vi "test Loopback with Disable.vi"(8 "error in":errorcluster, 11 "TestCase in":refnum<class "Single Core Simple Loopback.lvclass">) -> (0 "error out":errorcluster, 3 "TestCase out":refnum<class "Single Core Simple Loopback.lvclass">)   [LabVIEW 2020, in "Single Core Simple Loopback.lvclass"]
uses:
  Single Core Simple Loopback.lvclass
  C:/Git/niveristand-custom-device-testing-tools/VeriStandTestCase/VeriStandTestCase.lvclass
  <vilib>/numeric/Random Number (Range) I64.vi
  2771a990-9a12-45e1-bfa9-cf8078c77ee0.vi
  97c2081a-a4c0-4f2f-8a1c-7834fbf3da42.vi
  194ce8b8-c6d7-4123-a4fb-3c321acd640d.vi
  639b215b-9681-4d6c-ae13-b880b31cf4b5.vi
  <vilib>/numeric/sub_Random U32.vi
  <vilib>/NI VeriStand/Execution/Workspace/NI VeriStand - Get Single Channel Value.vi
  <vilib>/NI VeriStand/Execution/Workspace/NI VeriStand - Set Multiple Channel Values.vi
  <vilib>/NI VeriStand/Execution/Workspace/NI VeriStand - Get Multiple Channel Values.vi
  <vilib>/addons/_JKI Toolkits/VI Tester/TestCase.llb/TestCase.lvclass
  <vilib>/NI VeriStand/Execution/Workspace/NI_VS Workspace ExecutionAPI.lvlib
  niveristand-custom-device-testing-tools/VeriStandTestUtilities/VeriStandTestUtilities.lvlib
  C:/Program Files (x86)/National Instruments/LabVIEW 2020/vi.lib/addons/_JKI Toolkits/VI Tester/TestCase.llb/TestCase.lvclass
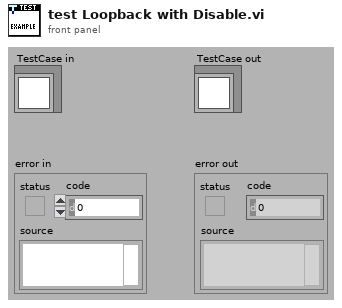
[diagram p1: front panel]
types:
  T1 = typedef "NI_VS Workspace ExecutionAPI.lvlib/WorkspaceAPI.ctl" = refnum<k24>
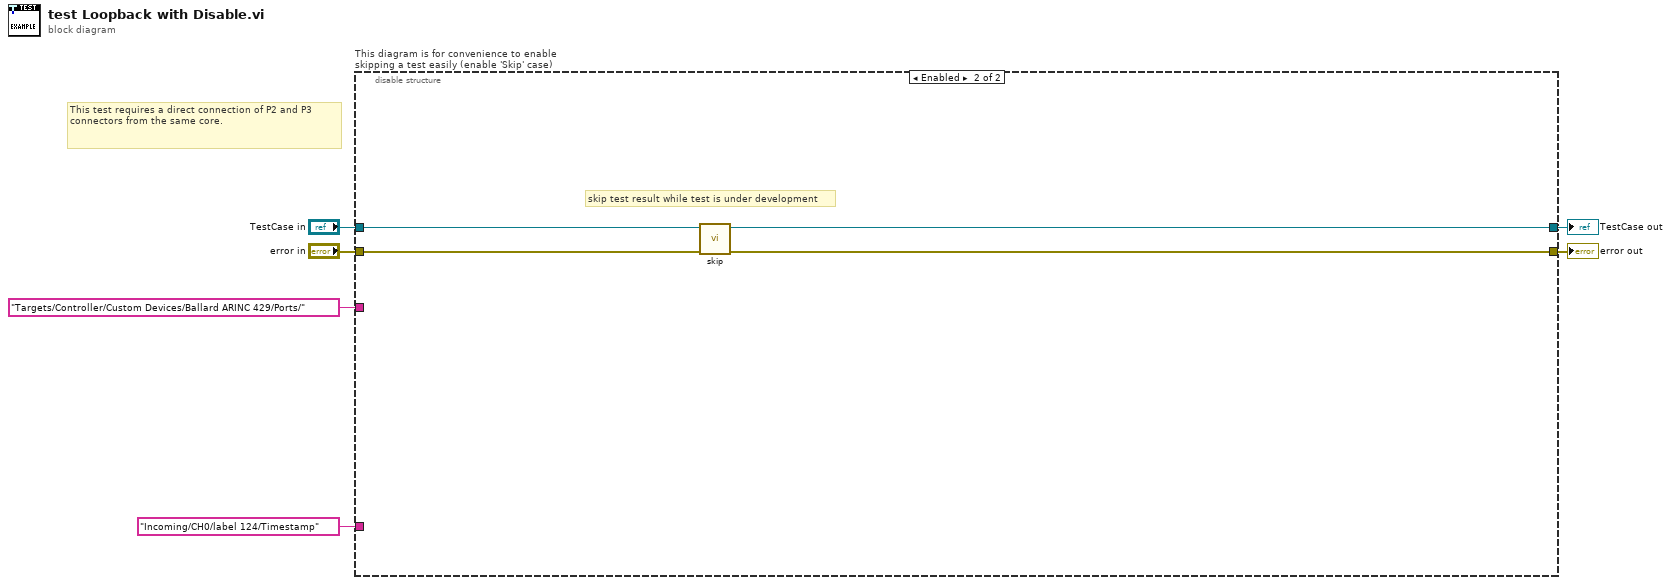
[diagram p0: block diagram]
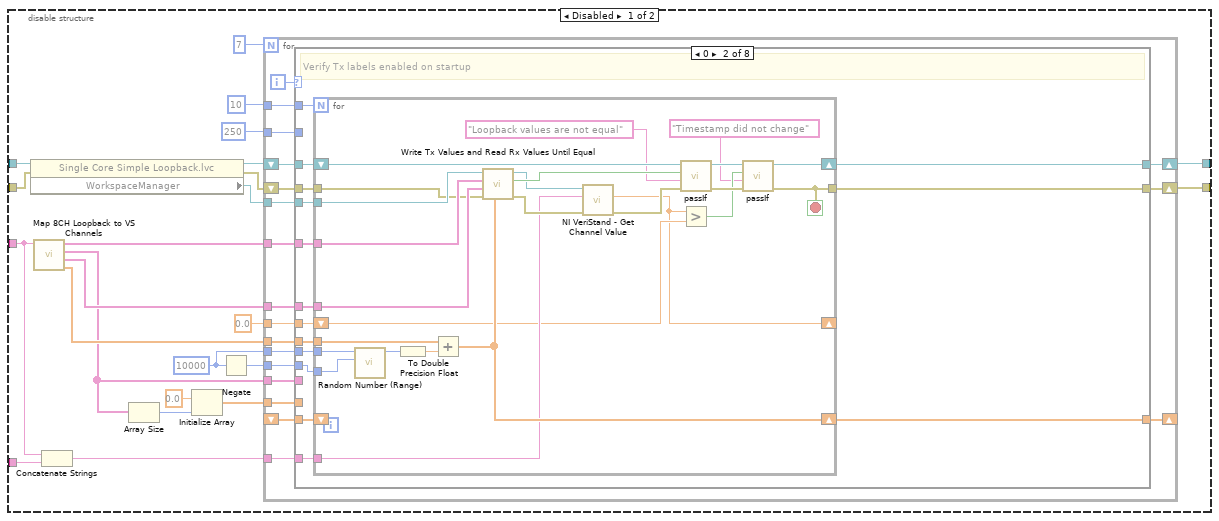
[diagram p2: hidden frame]
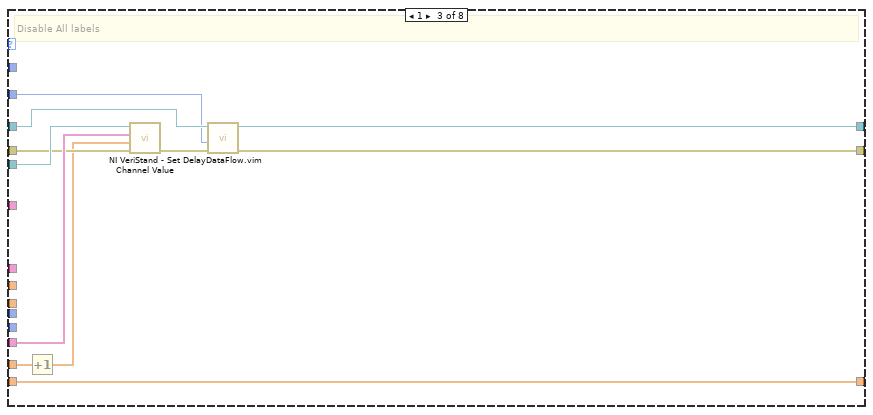
[diagram p4: hidden frame]
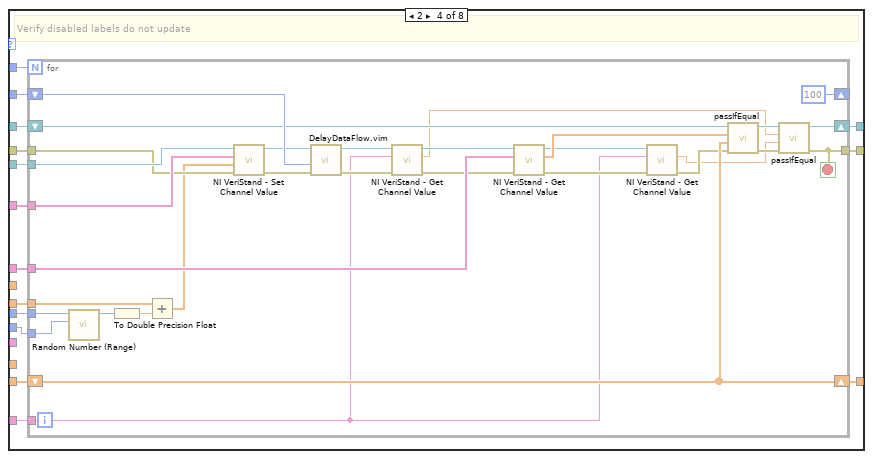
[diagram p5: hidden frame]
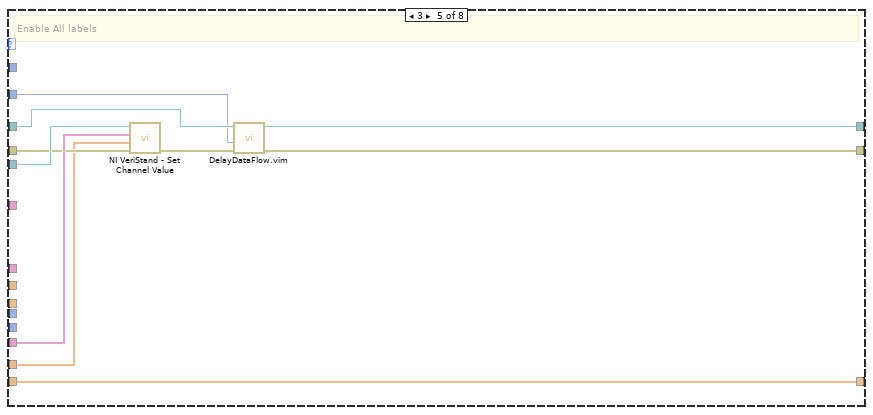
[diagram p6: hidden frame]
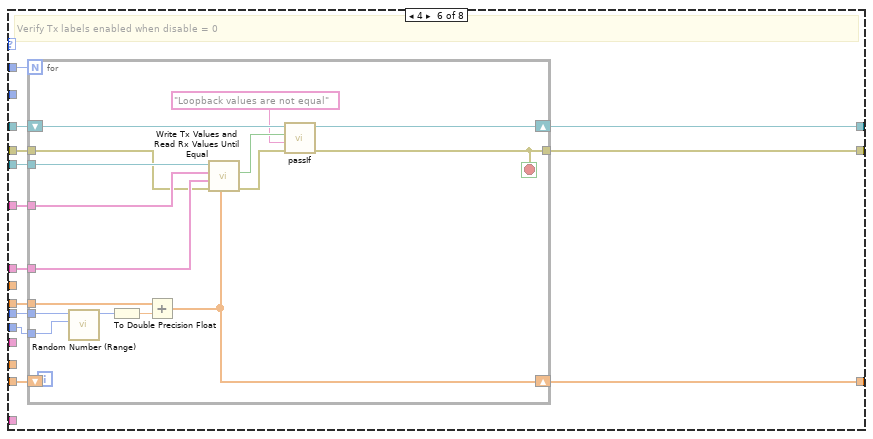
[diagram p7: hidden frame]
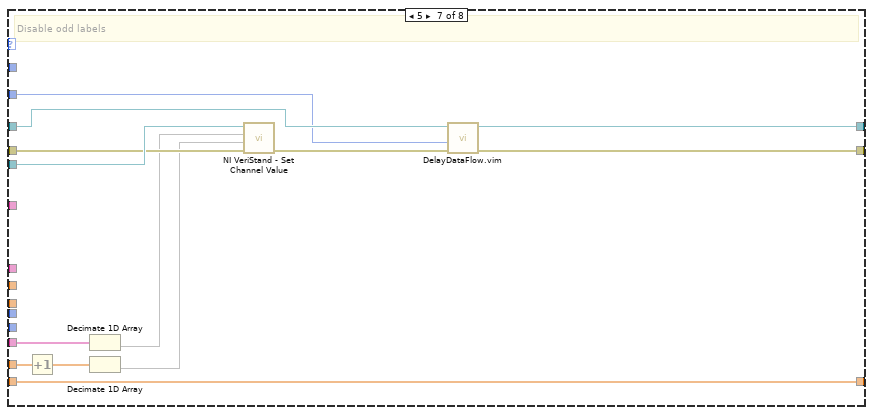
[diagram p8: hidden frame]
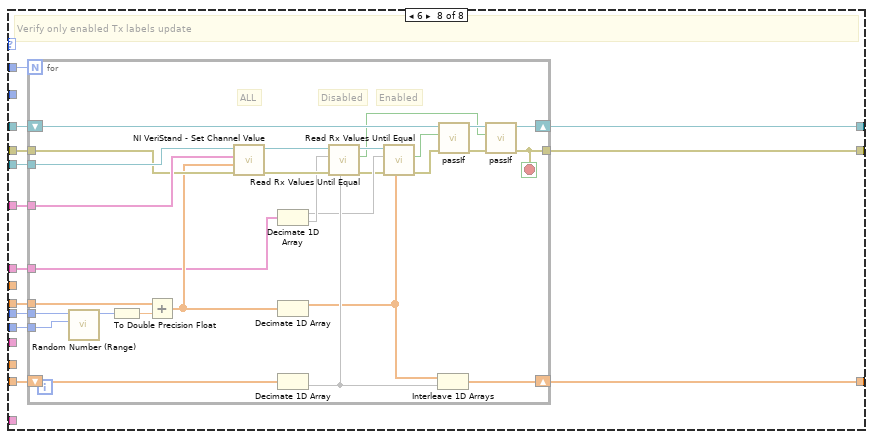
[diagram p9: hidden frame]
diagram:
  # "This test requires a direct connection of P2 and P3 connectors from the same core."
  n1 = disable-structure "This diagram is for convenience to enable skipping a test easily (enable 'Skip' case)" shown="Enabled" {
    disable-tunnel: "TestCase in" -> [w11 w241]
    disable-tunnel: [w8 w239] -> w3
    disable-tunnel: [w7 w240] -> w5
    disable-tunnel: "error in" -> [w10 w238]
    disable-tunnel: "Targets/Controller/Custom Devices/Ballard ARINC 429/Ports/" ("Channel") -> [w12 _]
    disable-tunnel: "Incoming/CH0/label 124/Timestamp" ("Channel") -> [w19 _]
    frame Disabled {
      w29 = i64 10000 ("upper bound (100)")
      n2 = property class="Single Core Simple Loopback.lvc"(reference=w11, error in=w10) -> (reference out=w25:refnum<class "Single Core Simple Loopback.lvclass">, error out=w9:errorcluster, "WorkspaceManager"=w27:T1)
      n3 = call "Map 8CH Loopback to VS Channels.vi"("Base Path to Ports"=w12) -> ("Channel Count"=w14:dbl[], "Rx Channel Array"=w15:string[], "Disable Channel Array"=w13:string[], "Tx Channel Array"=w16:string[])  [unwired: 7 in]
      n4 = Concatenate Strings(w12, w19) -> (w18:string)
      n5 = Array Size(array=w13) -> (size(s)=w24:i32)
      n6 = Initialize Array(0.0 ("element"), w24) -> (w22:dbl[])
      n7 = Negate(x=w29) -> (-x=w28:i64)
      n8 = for {
        N: 7 -> [_]
        tunnel: w14 -> [w48]
        tunnel: w29 -> [w47]
        tunnel: w28 -> [w46]
        tunnel: w16 -> [w45]
        tunnel: w27 -> [w44]
        tunnel: 10 -> [w43]
        tunnel: w15 -> [w41]
        shift-right: [w38] -> w7
        shift-left: w9 -> [w42]
        shift-right: [w39] -> w8
        shift-left: w25 -> [w40]
        tunnel: w13 -> [w36]
        tunnel: w22 -> [w35]
        shift-right: [w34] -> _
        shift-left: _ -> [w33]
        tunnel: u32 250 ("milliseconds to wait") -> [w32]
        tunnel: w18 -> [w31]
        tunnel: 0.0 ("Value") -> [w30]
        i -> [w37]
        n9 = case shown="0" w37 {
          tunnel: w48 -> [_ w66 _ w116 _ w168 _ w209]
          tunnel: w47 -> [_ w65 _ w115 _ w167 _ w208]
          tunnel: w46 -> [_ w64 _ w114 _ w166 _ w207]
          tunnel: w45 -> [_ w63 _ w113 _ w165 _ w206]
          tunnel: w44 -> [_ w62 w101 w112 w155 w164 w196 w205]
          tunnel: w43 -> [_ w61 _ w111 _ w163 _ w204]
          tunnel: w42 -> [w50 w60 w99 w110 w153 w162 w195 w203]
          tunnel: w41 -> [_ w59 _ w109 _ w161 _ w202]
          tunnel: w40 -> [w51 w58 w97 w108 w152 w160 w193 w201]
          tunnel: [w51 w57 w97 w107 w152 w159 w193 w200] -> w39
          tunnel: [w50 w56 w96 w106 w150 w158 w192 w199] -> w38
          tunnel: w36 -> [_ _ w100 _ w154 _ w187 _]
          tunnel: w35 -> [_ _ w98 _ w148 _ w194 _]
          tunnel: [w49 w55 w95 w104 w149 w157 w191 w198] -> w34
          tunnel: w33 -> [w49 w54 w95 w105 w149 w156 w191 w197]
          tunnel: w32 -> [_ _ w92 w103 w147 _ w185 _]
          tunnel: w31 -> [_ w53 _ w102 _ _ _ _]
          tunnel: w30 -> [_ w52 _ _ _ _ _ _]
          frame Default {
          }
          frame 0 {
            # "Verify Tx labels enabled on startup"
            n10 = for {
              N: w61 -> [_]
              tunnel: w66 -> [w89]
              tunnel: w65 -> [w88]
              tunnel: w64 -> [w87]
              tunnel: w63 -> [w84]
              tunnel: w62 -> [w85]
              tunnel: w60 -> [w81]
              tunnel: w59 -> [w83]
              shift-right: [w72] -> w57
              shift-left: w58 -> [w86]
              tunnel: [w73] -> w56
              shift-right: [w82] -> w55
              shift-left: w54 -> [_]
              tunnel: w53 -> [w77]
              shift-right: [w70] -> _
              shift-left: w52 -> [w71]
              stop <- w73 stop-if-true
              n11 = call-poly <vilib>:"Random Number (Range).vi"("lower bound (-100)"=w87, "upper bound (100)"=w88) -> ("number"=w91:i64)  [unwired: 9 in]
              n12 = To Double Precision Float(number=w91) -> (double precision float=w90:dbl)
              n13 = Add(x=w89, y=w90) -> (x+y=w82:dbl[])
              n14 = call "Write Tx Values and Read Rx Values Until Equal.vi"("Tx values"=w82, "error in"=w81, "Rx aliases"=w83, "Tx aliases"=w84, "workspace manager in"=w85) -> ("error out"=w79:errorcluster, "values equal"=w80:bool, "workspace manager out"=w76:T1)  [unwired: 4 in]
              n15 = call-poly <vilib>:"NI VeriStand - Get Channel Value.vi"("error in (no error)"=w79, "Channel"=w77, "WorkspaceManager in"=w76) -> ("error out"=w78:errorcluster, "Value"=w70:dbl)  [unwired: 6 in, 1 out]
              n16 = call-dynamic "passIf.vi"("error in (no error)"=w78, "message (\"\")"="Loopback values are not equal" ("message (\"\")"), "pass"=w80, "TestCase in"=w86) -> ("error out"=w74:errorcluster, "TestCase out"=w75:refnum<class "Single Core Simple Loopback.lvclass">)  [unwired: 6 in]
              n17 = Greater?(x=w70, y=w71) -> (0:w69:bool)
              n18 = call-dynamic "passIf.vi"("error in (no error)"=w74, "message (\"\")"="Timestamp did not change" ("message (\"\")"), "pass"=w69, "TestCase in"=w75) -> ("error out"=w73:errorcluster, "TestCase out"=w72:refnum<class "Single Core Simple Loopback.lvclass">)  [unwired: 6 in]
            }
          }
          frame 1 {
            # "Disable All labels"
            n19 = Increment(x=w98) -> (x+1=w94:dbl[])
            n20 = call-poly <vilib>:"NI VeriStand - Set Channel Value.vi"("error in (no error)"=w99, "Values"=w94, "Channels"=w100, "WorkspaceManager in"=w101) -> ("error out"=w93:errorcluster)  [unwired: 6 in, 1 out]
            n21 = call "DelayDataFlow.vim"("value in"=w93, "milliseconds to wait"=w92) -> ("value out"=w96:errorcluster)  [unwired: 2 in, 1 out]
          }
          frame 2 {
            # "Verify disabled labels do not update"
            n22 = for {
              N: w111 -> [_]
              tunnel: w116 -> [w143]
              tunnel: w115 -> [w142]
              tunnel: w114 -> [w141]
              tunnel: w113 -> [w140]
              tunnel: w112 -> [w139]
              tunnel: w110 -> [w137]
              tunnel: w109 -> [w136]
              shift-right: [w120] -> w107
              shift-left: w108 -> [w135]
              tunnel: [w119] -> w106
              shift-right: [w132] -> w104
              shift-left: w105 -> [w132]
              shift-right: [u32 100 ("milliseconds to wait")] -> _
              shift-left: w103 -> [w138]
              tunnel: w102 -> [w124]
              stop <- w119 stop-if-true
              n23 = call-poly <vilib>:"Random Number (Range).vi"("lower bound (-100)"=w141, "upper bound (100)"=w142) -> ("number"=w145:i64)  [unwired: 9 in]
              n24 = To Double Precision Float(number=w145) -> (double precision float=w144:dbl)
              n25 = Add(x=w143, y=w144) -> (x+y=w133:dbl[])
              n26 = call-poly <vilib>:"NI VeriStand - Set Channel Value.vi"("error in (no error)"=w137, "Values"=w133, "Channels"=w140, "WorkspaceManager in"=w139) -> ("error out"=w146:errorcluster, "WorkspaceManager out"=w130:T1)  [unwired: 6 in]
              n27 = call "DelayDataFlow.vim"("value in"=w146, "milliseconds to wait"=w138) -> ("value out"=w129:errorcluster)  [unwired: 2 in, 1 out]
              n28 = call-poly <vilib>:"NI VeriStand - Get Channel Value.vi"("error in (no error)"=w129, "Channel"=w124, "WorkspaceManager in"=w130) -> ("error out"=w128:errorcluster, "Value"=w117:dbl, "WorkspaceManager out"=w127:T1)  [unwired: 6 in]
              n29 = call-poly <vilib>:"NI VeriStand - Get Channel Value.vi"("error in (no error)"=w128, "Channels"=w136, "WorkspaceManager in"=w127) -> ("error out"=w126:errorcluster, "Values"=w134:dbl[], "WorkspaceManager out"=w125:T1)  [unwired: 6 in]
              n30 = call-poly <vilib>:"NI VeriStand - Get Channel Value.vi"("error in (no error)"=w126, "Channel"=w124, "WorkspaceManager in"=w125) -> ("error out"=w123:errorcluster, "Value"=w118:dbl)  [unwired: 6 in, 1 out]
              n31 = call-dynamic "passIfEqual.vi"("error in (no error)"=w123, "y"=w132, "x"=w134, "TestCase in"=w135) -> ("error out"=w121:errorcluster, "TestCase out"=w122:refnum<class "Single Core Simple Loopback.lvclass">)  [unwired: 6 in]
              n32 = call-dynamic "passIfEqual.vi"("error in (no error)"=w121, "y"=w118, "x"=w117, "TestCase in"=w122) -> ("error out"=w119:errorcluster, "TestCase out"=w120:refnum<class "Single Core Simple Loopback.lvclass">)  [unwired: 6 in]
            }
          }
          frame 3 {
            # "Enable All labels"
            n33 = call-poly <vilib>:"NI VeriStand - Set Channel Value.vi"("error in (no error)"=w153, "Values"=w148, "Channels"=w154, "WorkspaceManager in"=w155) -> ("error out"=w151:errorcluster)  [unwired: 6 in, 1 out]
            n34 = call "DelayDataFlow.vim"("value in"=w151, "milliseconds to wait"=w147) -> ("value out"=w150:errorcluster)  [unwired: 2 in, 1 out]
          }
          frame 4 {
            # "Verify Tx labels enabled when disable = 0"
            n35 = for {
              N: w163 -> [_]
              tunnel: w168 -> [w182]
              tunnel: w167 -> [w181]
              tunnel: w166 -> [w180]
              tunnel: w165 -> [w175]
              tunnel: w164 -> [w176]
              tunnel: w162 -> [w172]
              tunnel: w161 -> [w174]
              shift-right: [w178] -> w159
              shift-left: w160 -> [w179]
              tunnel: [w177] -> w158
              shift-right: [w173] -> w157
              shift-left: w156 -> [_]
              stop <- w177 stop-if-true
              n36 = call-poly <vilib>:"Random Number (Range).vi"("lower bound (-100)"=w180, "upper bound (100)"=w181) -> ("number"=w184:i64)  [unwired: 9 in]
              n37 = To Double Precision Float(number=w184) -> (double precision float=w183:dbl)
              n38 = Add(x=w182, y=w183) -> (x+y=w173:dbl[])
              n39 = call "Write Tx Values and Read Rx Values Until Equal.vi"("Tx values"=w173, "error in"=w172, "Rx aliases"=w174, "Tx aliases"=w175, "workspace manager in"=w176) -> ("error out"=w171:errorcluster, "values equal"=w170:bool)  [unwired: 4 in, 1 out]
              n40 = call-dynamic "passIf.vi"("error in (no error)"=w171, "message (\"\")"="Loopback values are not equal" ("message (\"\")"), "pass"=w170, "TestCase in"=w179) -> ("error out"=w177:errorcluster, "TestCase out"=w178:refnum<class "Single Core Simple Loopback.lvclass">)  [unwired: 6 in]
            }
          }
          frame 5 {
            # "Disable odd labels"
            n41 = Increment(x=w194) -> (x+1=w188:dbl[])
            n42 = Decimate 1D Array(w187) -> (w189:string[])  [unwired: 1 out]
            n43 = Decimate 1D Array(w188) -> (w186:dbl[])  [unwired: 1 out]
            n44 = call-poly <vilib>:"NI VeriStand - Set Channel Value.vi"("error in (no error)"=w195, "Values"=w186, "Channels"=w189, "WorkspaceManager in"=w196) -> ("error out"=w190:errorcluster)  [unwired: 6 in, 1 out]
            n45 = call "DelayDataFlow.vim"("value in"=w190, "milliseconds to wait"=w185) -> ("value out"=w192:errorcluster)  [unwired: 2 in, 1 out]
          }
          frame 6 {
            # "Verify only enabled Tx labels update"
            n46 = for {
              N: w204 -> [_]
              tunnel: w209 -> [w235]
              tunnel: w208 -> [w234]
              tunnel: w207 -> [w233]
              tunnel: w206 -> [w232]
              tunnel: w205 -> [w231]
              tunnel: w203 -> [w230]
              tunnel: w202 -> [w220]
              shift-right: [w229] -> w200
              shift-left: w201 -> [w223]
              tunnel: [w228] -> w199
              shift-right: [w225] -> w198
              shift-left: w197 -> [w226]
              stop <- w228 stop-if-true
              # "Enabled"
              # "Disabled"
              # "ALL"
              n47 = call-poly <vilib>:"Random Number (Range).vi"("lower bound (-100)"=w233, "upper bound (100)"=w234) -> ("number"=w237:i64)  [unwired: 9 in]
              n48 = To Double Precision Float(number=w237) -> (double precision float=w236:dbl)
              n49 = Add(x=w235, y=w236) -> (x+y=w227:dbl[])
              n50 = call-poly <vilib>:"NI VeriStand - Set Channel Value.vi"("error in (no error)"=w230, "Values"=w227, "Channels"=w232, "WorkspaceManager in"=w231) -> ("error out"=w221:errorcluster, "WorkspaceManager out"=w224:T1)  [unwired: 6 in]
              n51 = Decimate 1D Array(w220) -> (w216:string[], w219:string[])
              n52 = Decimate 1D Array(w227) -> (w215:dbl[])  [unwired: 1 out]
              n53 = Decimate 1D Array(w226) -> (w218:dbl[])  [unwired: 1 out]
              n54 = call "Read Rx Values Until Equal.vi"("expected values"=w218, "error in"=w221, "Rx aliases"=w219, "workspace manager in"=w224) -> ("error out"=w214:errorcluster, "values equal expected"=w210:bool, "workspace manager out"=w217:T1)  [unwired: 5 in]
              n55 = call "Read Rx Values Until Equal.vi"("expected values"=w215, "error in"=w214, "Rx aliases"=w216, "workspace manager in"=w217) -> ("error out"=w213:errorcluster, "values equal expected"=w211:bool)  [unwired: 5 in, 1 out]
              n56 = Interleave 1D Arrays(w215, w218) -> (w225:dbl[])
              n57 = call-dynamic "passIf.vi"("error in (no error)"=w213, "pass"=w211, "TestCase in"=w223) -> ("error out"=w212:errorcluster, "TestCase out"=w222:refnum<class "Single Core Simple Loopback.lvclass">)  [unwired: 7 in]
              n58 = call-dynamic "passIf.vi"("error in (no error)"=w212, "pass"=w210, "TestCase in"=w222) -> ("error out"=w228:errorcluster, "TestCase out"=w229:refnum<class "Single Core Simple Loopback.lvclass">)  [unwired: 7 in]
            }
          }
        }
      }
    }
    frame Enabled {
      # "skip test result while test is under development"
      n59 = call <vilib>:"skip.vi"("error in (no error)"=w238, "TestCase in"=w241) -> ("error out"=w240:errorcluster, "TestCase out"=w239:refnum<class "Single Core Simple Loopback.lvclass">)  [unwired: 8 in]
    }
  }
  "error out" <- w5
  "TestCase out" <- w3
